vi "Enqueue MHL Queue-array.vi"(7 "Add to front? (dflt = F)":bool[](array[boolean]), 8 "error in (no error)":errorcluster, 10 "Array of data (dflt=empty)":variant[](array[variant]), 11 "Commands":string[](array[string])) -> (0 "error out":errorcluster)   [LabVIEW 2020, in "main.lvlib"]
doc: "Blank VI with error handling."
uses:
  main.lvlib
  PTRL/errors/errors.lvlib
panel:
  out "Loop iteration":i32
  out "\"Add to front\" size-after":i32
  out "\"Add to front\" size-before":i32
  out "Variant Data size-after":i32
  out "Variant Data size-before":i32
  out "Commands size":i32
  # "Development\ncontrols/indicators useful for development and testing, but which are not outputs of the VI"
  # "Input\nInputs to the VI"
  # "Output\nOutputs of the VI"
  # "Description\n\nBlank VI with error handling case. \n\nSummarize the use of this VI in this space."
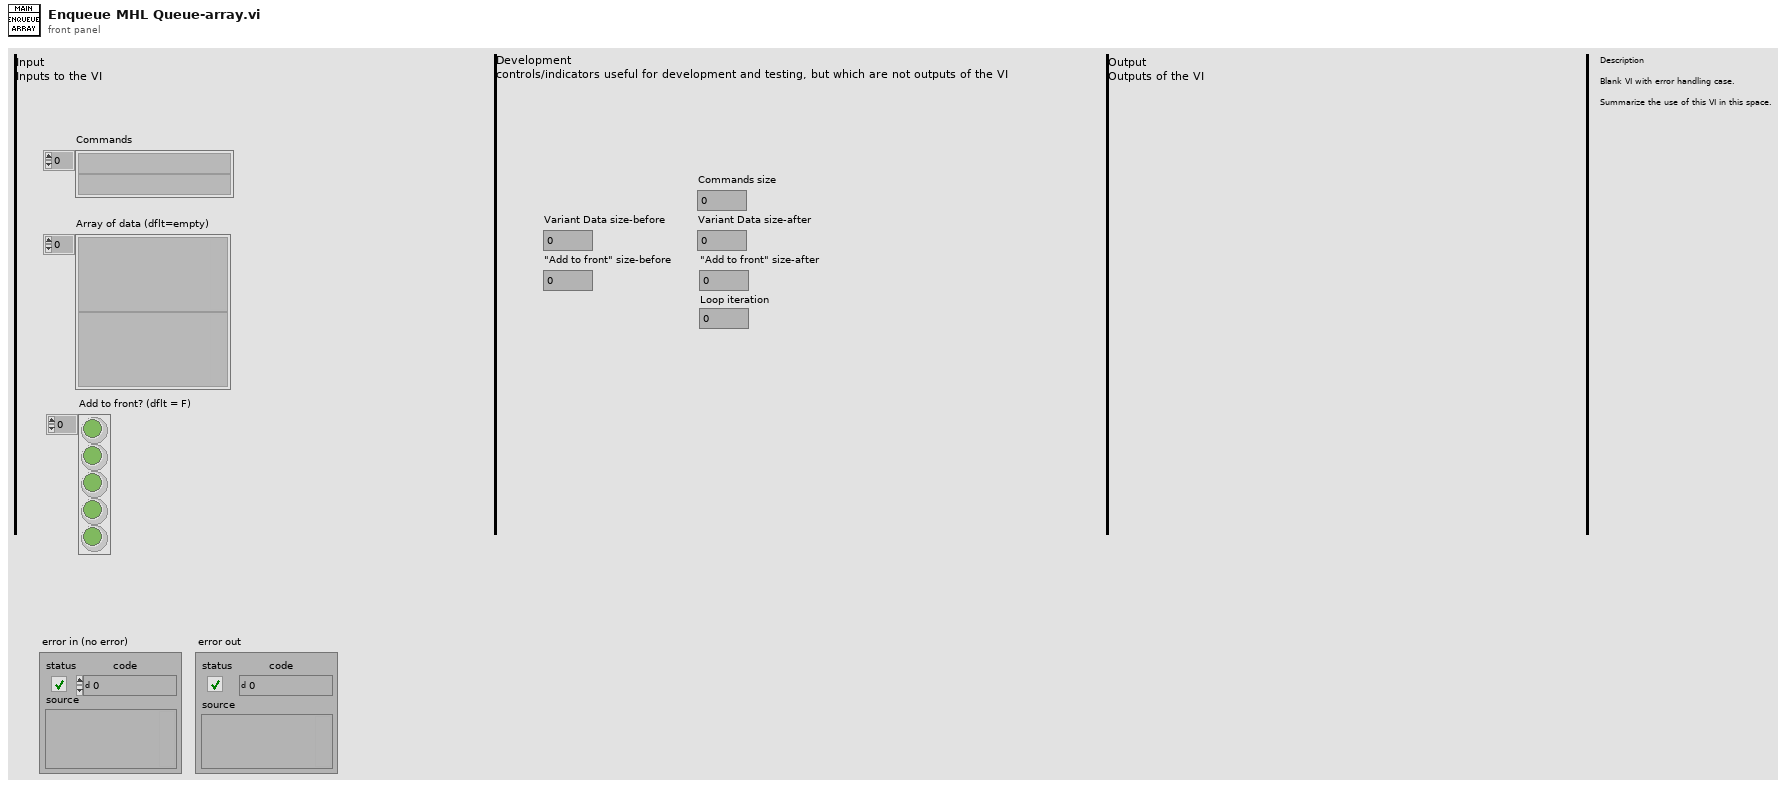
[diagram p1: front panel]
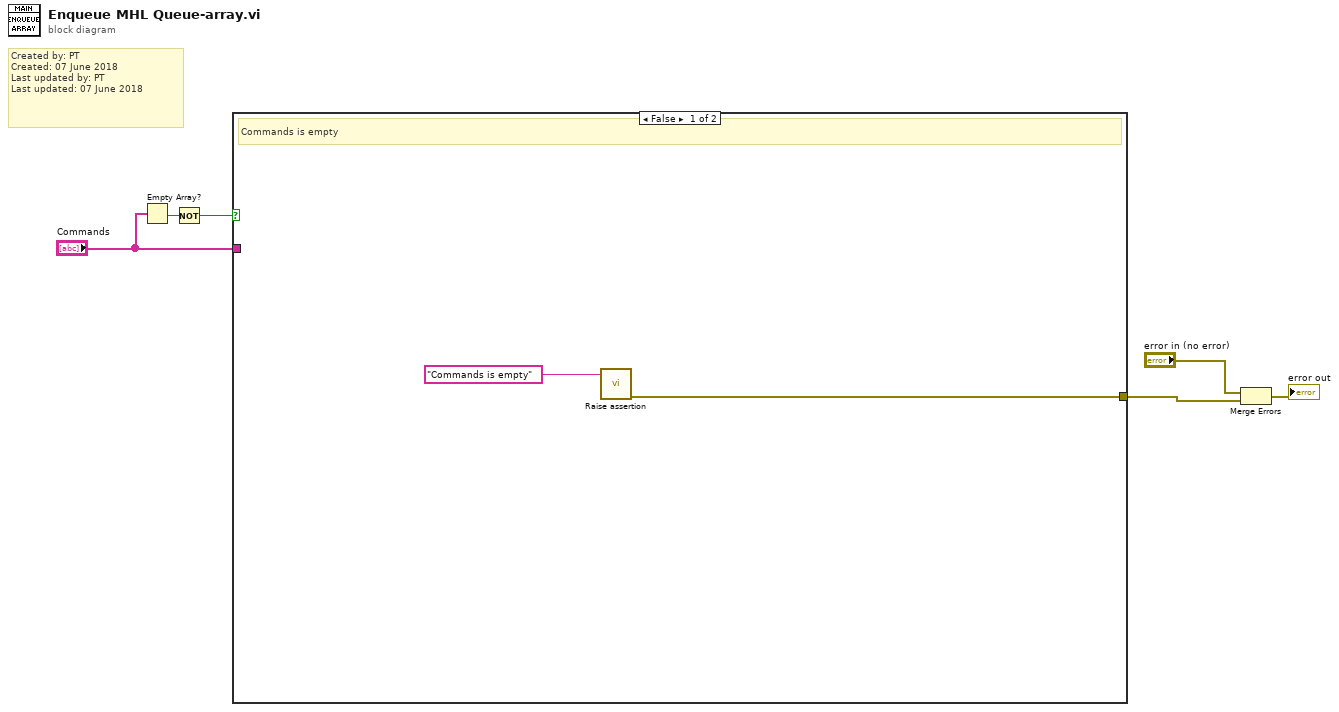
[diagram p0: block diagram]
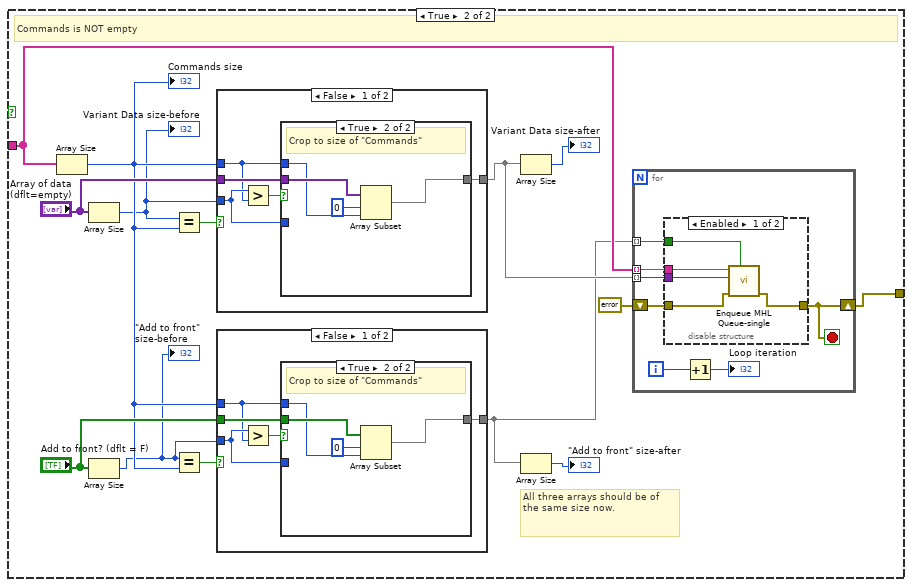
[diagram p2: hidden frame]
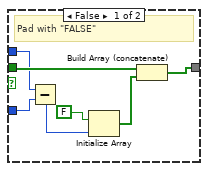
[diagram p4: hidden frame]
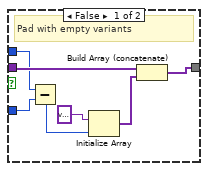
[diagram p6: hidden frame]
diagram:
  # "Created by: PT\nCreated: 07 June 2018\nLast updated by: PT\nLast updated: 07 June 2018"
  n1 = Empty Array?(array="Commands") -> (empty?=w4:bool)
  n2 = Not(x=w4) -> (.not. x?=w3:bool)
  n3 = case shown="False" w3 {
    tunnel: "Commands" -> [_ w13]
    tunnel: [w7 w9] -> w1
    frame False {
      # "Commands is empty"
      n4 = call "Raise assertion.vi"("Details (dflt=\"no details\")"="Commands is empty") -> ("error out"=w7:errorcluster)  [unwired: 10 in]
    }
    frame True {
      # "All three arrays should be of the same size now."
      # "Commands is NOT empty"
      n5 = Array Size(array=w13) -> (size(s)=w18:i32)
      "Commands size" <- w18
      n6 = Array Size(array="Array of data (dflt=empty)") -> (size(s)=w17:i32)
      "Variant Data size-before" <- w17
      n7 = Array Size(array="Add to front? (dflt = F)") -> (size(s)=w15:i32)
      "\"Add to front\" size-before" <- w15
      n8 = Equal?(x=w17, y=w18) -> (x = y?=w22:bool)
      n9 = Equal?(x=w15, y=w18) -> (x = y?=w20:bool)
      n10 = case shown="False" w22 {
        tunnel: "Array of data (dflt=empty)" -> [w56 w69]
        tunnel: [w54 w69] -> w12
        tunnel: w18 -> [w53 _]
        tunnel: w17 -> [w55 _]
        frame False {
          n11 = Greater?(x=w55, y=w53) -> (0:w57:bool)
          n12 = case shown="True" w57 {
            tunnel: w56 -> [w63 w68]
            tunnel: w55 -> [w60 _]
            tunnel: [w58 w66] -> w54
            tunnel: w53 -> [w61 w65]
            frame False {
              # "Pad with empty variants"
              n13 = Subtract(x=w61, y=w60) -> (x-y=w59:i32)
              n14 = Initialize Array(variant, w59) -> (w62:variant[])
              n15 = Build Array (concatenate)(w63, w62) -> (w58:variant[])
            }
            frame True {
              # "Crop to size of \"Commands\""
              n16 = Array Subset(array=w68, index=0, length=w65) -> (w66:variant[])
            }
          }
        }
        frame True {
        }
      }
      n17 = case shown="False" w20 {
        tunnel: "Add to front? (dflt = F)" -> [w39 w52]
        tunnel: [w37 w52] -> w11
        tunnel: w18 -> [w36 _]
        tunnel: w15 -> [w38 _]
        frame False {
          n18 = Greater?(x=w38, y=w36) -> (0:w40:bool)
          n19 = case shown="True" w40 {
            tunnel: w39 -> [w46 w51]
            tunnel: w38 -> [w43 _]
            tunnel: [w41 w49] -> w37
            tunnel: w36 -> [w44 w48]
            frame False {
              # "Pad with \"FALSE\""
              n20 = Subtract(x=w44, y=w43) -> (x-y=w42:i32)
              n21 = Initialize Array(FALSE, w42) -> (w45:bool[])
              n22 = Build Array (concatenate)(w46, w45) -> (w41:bool[])
            }
            frame True {
              # "Crop to size of \"Commands\""
              n23 = Array Subset(array=w51, index=0, length=w48) -> (w49:bool[])
            }
          }
        }
        frame True {
        }
      }
      n24 = Array Size(array=w12) -> (size(s)=→"Variant Data size-after":i32)
      n25 = Array Size(array=w11) -> (size(s)=→"\"Add to front\" size-after":i32)
      n26 = for {
        tunnel: w13 -> [w29] mode=indexing
        tunnel: w12 -> [w28] mode=indexing
        tunnel: w11 -> [w27] mode=indexing
        shift-right: [w23] -> w9
        shift-left: errorcluster {"status"=FALSE, "code"=0, "source"=""} ("error constant") -> [w26]
        i -> [w25]
        stop <- w23 stop-if-true
        n27 = disable-structure shown="Enabled" {
          disable-tunnel: w29 -> [w31 _]
          disable-tunnel: w28 -> [w30 _]
          disable-tunnel: w27 -> [w34 _]
          disable-tunnel: w26 -> [w33 w35]
          disable-tunnel: [w32 w35] -> w23
          frame Enabled {
            n28 = call "Enqueue MHL Queue-single.vi"("Add To Front (F)"=w34, "ErrorIn"=w33, "Data"=w30, "Command"=w31) -> ("ErrorOut"=w32:errorcluster)  [unwired: 7 in]
          }
          frame Disabled {
          }
        }
        n29 = Increment(x=w25) -> (x+1=→"Loop iteration":i32)
      }
    }
  }
  n30 = Merge Errors("error in (no error)", w1) -> (→"error out":errorcluster)
